vi "Filter Control Mouse Down Event.vi"(8 "error in (no error)":errorcluster, 10 "ControlMouseDownMsg":refnum<class "ControlMouseDownMsg.lvclass">, 11 "GarphEventFilter in":refnum<class "GarphEventFilter.lvclass">) -> (0 "error out":errorcluster, 1 "Discard?":bool, 2 "Filtered Event Data":T1, 3 "GarphEventFilter out":refnum<class "GarphEventFilter.lvclass">, 5 "Data Filtered?":bool)   [LabVIEW 2020, in "GarphView.lvlib" / "GarphEventFilter.lvclass"]
uses:
  GarphEventFilter.lvclass
  GarphEventFilter.lvclass/GarphEventFilter.ctl
  <vilib>/gpm_packages/@cs/mva-viewable/Source/ActorEvents/IEventAggregator Messages/ControlMouseDownMsg/ControlMouseDownMsg.lvclass
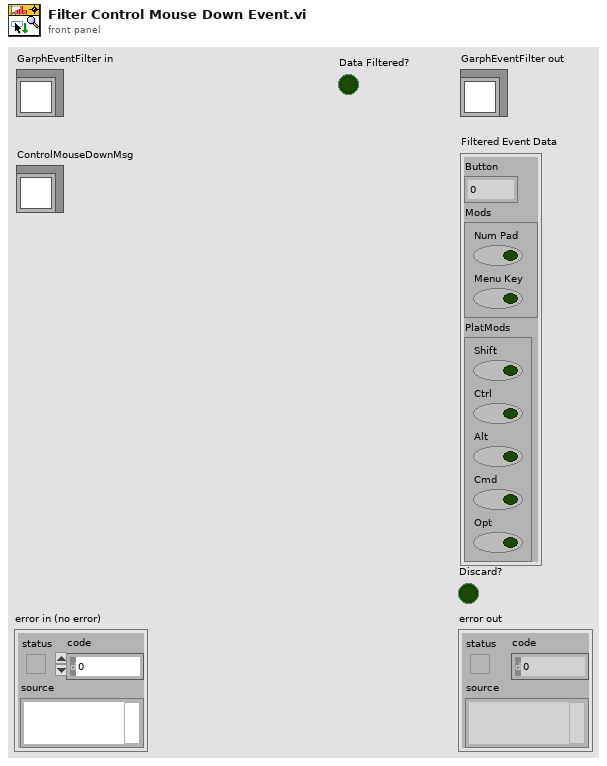
[diagram p1: front panel]
types:
  T1 = cluster{"Button":u16, "Mods":cluster{"Num Pad":bool, "Menu Key":bool}, "PlatMods":cluster{"Shift":bool, "Ctrl":bool, "Alt":bool, "Cmd":bool, "Opt":bool}}
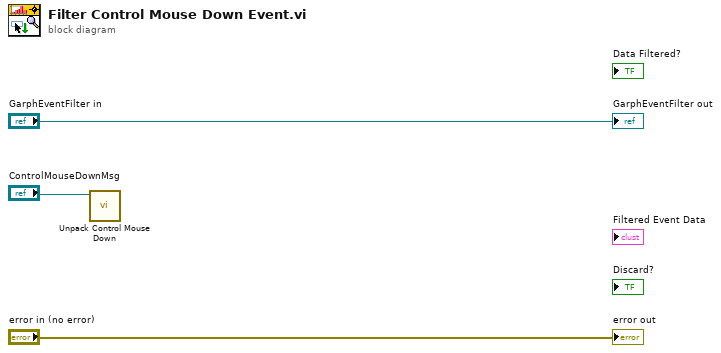
[diagram p0: block diagram]
diagram:
  n1 = call <vilib>:"Unpack Control Mouse Down.vi"("ControlMouseDownMsg"="ControlMouseDownMsg") -> ()  [unwired: 4 in, 7 out]
  "error out" <- "error in (no error)"
  "GarphEventFilter out" <- "GarphEventFilter in"
